vi "BRig_dataBlock_init.vi"() -> (0 "output_nCol":i32=33, 3 "output_dataBlock":u16[][](array[numeric]))   [LabVIEW 2014]
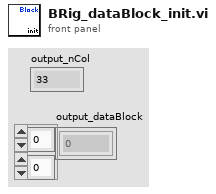
[diagram p1: front panel]
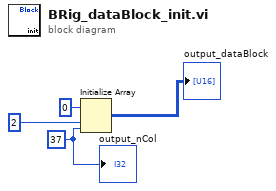
[diagram p0: block diagram]
diagram:
  w1 = 37 ("dimension size")
  n1 = Initialize Array(u16 0 ("element"), 2 ("dimension size"), w1) -> (→"output_dataBlock":u16[][])
  "output_nCol" <- w1
